vi "PTScanner.set central values.vi"(0 "i ref in":refnum<vi>, 5 "error in(no error)":errorcluster) -> (14 "i ref out":refnum<vi>, 19 "error out":errorcluster)   [LabVIEW 2014, in "PTScanner.lvlib"]
uses:
  PTScanner.lvlib
  CS_Core/CSSystem/CSSystemLib/CSSystemLib.lvlib
  CS_Core/BaseProcess/BaseProcess.lvlib
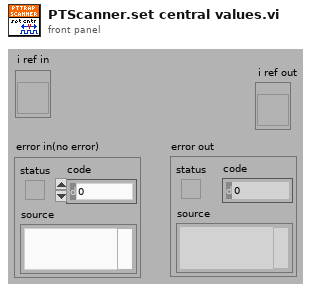
[diagram p1: front panel]
types:
  T1 = typedef "PTScanner.lvlib/PTScanner.i attribute.ctl" = cluster{"Object cmds":T2[], "Steps":cluster{"Finished":bool, "cmd setup":T3[]}[], "curStep":i32, "DIM IDs":cluster{"AllFinished":i32, "Finished":i32, "curStep":i32, "nofSteps":i32, "NomValues":i32[], "1D-Min":i32, "1D-Max":i32, "Dimensions":i32, "MaxDimensions":i32, "ScanedDeviceNames":i32[]}, "All Finished":bool, "DIMs in use":string[], "Running":bool, "Scan Delay":u32, "loop":bool, "Paused":bool, "Formed":bool}
  T2 = typedef "PTScanner.lvlib/PTScanner.obj parameters.ctl" = cluster{"object":string, "DIM address":string, "method":string, "data descriptor":string, "method parameters":cluster{"Name":string, "Descr":string, "Value":string, "Value?":bool}[], "Call Mode":enum16{"Simple DIM", "Synchronous"}, "actValue":dbl, "Centroid":dbl, "Minus Delta":dbl, "Plus Delta":dbl, "increment":dbl, "DIM Status":cluster{"no link":bool, "quality":i32, "Time Stamp":timestamp}, "range":dbl, "DIMChannelIndex":i32}
  T3 = typedef "PTScanner.lvlib/PTScanner.step obj parameters.ctl" = cluster{"obj index":i32, "nomValue":dbl, "fulfilled":bool}
  T4 = cluster{"Name":string, "Descr":string, "Value":string, "Value?":bool}[]
  T5 = typedef "CoreDefs.rawDataType.ctl" = i8[]
  T6 = typedef "CoreDefs.call_type.ctl" = cluster{"Object":string, "Selector":string, "CallType":enum16{"simple", "synchronous", "asynchronous"}, "Async Object":string, "Async Selector":string, "Data Descriptor":T7, "Data":T5, "Error #":i32, "Expire":u32}
  T7 = typedef "BaseProcess.lvlib/BaseProcess.descriptor string definition.ctl" = string
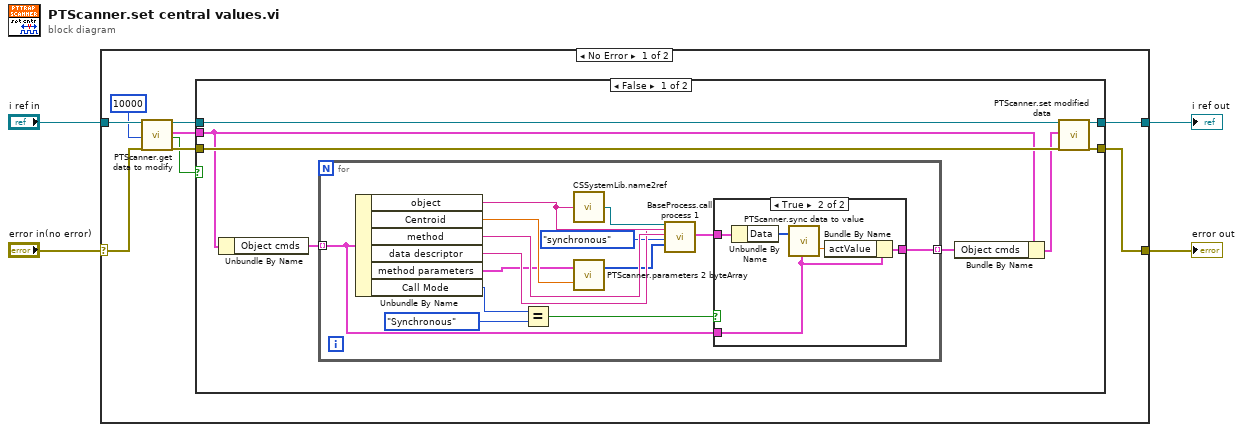
[diagram p0: block diagram]
diagram:
  n1 = case shown="No Error" "error in(no error)" {
    selector: "error in(no error)" -> [w12 w44]
    tunnel: [w8 w44] -> w3
    tunnel: [w9 w45] -> w2
    tunnel: "i ref in" -> [w13 w45]
    frame No Error {
      n2 = call "PTScanner.get data to modify.vi"("i ref in"=w13, "ms timeout (10000)"=10000, "error in (no error)"=w12) -> ("i ref out"=w10:refnum<vi>, "i attribute"=w7:T1, "timed out"=w6:bool, "error out"=w11:errorcluster)  [unwired: 13 in]
      n3 = case shown="False" w6 {
        tunnel: w11 -> [w20 w42]
        tunnel: w10 -> [w19 w43]
        tunnel: [w18 w43] -> w9
        tunnel: [w17 w42] -> w8
        tunnel: w7 -> [w15 _]
        frame False {
          n4 = Unbundle By Name(w15) -> ("Object cmds"=w21:T2[])
          n5 = for {
            tunnel: w21 -> [w22] mode=indexing
            tunnel: [w23] -> w16 mode=indexing
            n6 = Unbundle By Name(w22) -> ("object"=w34:string, "Centroid"=w30:dbl, "method"=w33:string, "data descriptor"=w32:string, "method parameters"=w27:T4, "Call Mode"=w26:enum16{"Simple DIM", "Synchronous"})
            n7 = Equal?(x=w26, y=enum16{"Simple DIM", "Synchronous"}."Synchronous" ("Call Mode")) -> (x = y?=w24:bool)
            n8 = call "CSSystemLib.name2ref.vi"("name"=w34) -> ("obj refnum"=w35:refnum<vi>)
            n9 = call "PTScanner.parameters 2 byteArray.vi"("Parameters"=w27, "nomValue"=w30) -> ("byteArray out"=w29:T5)  [unwired: 17 in]
            n10 = call "BaseProcess.call process 1.vi"("i ref in"=w35, "Object"=w34, "Selector"=w33, "CallType"=enum16{"simple", "synchronous", "asynchronous"}."synchronous", "Data"=w29, "Data Descriptor"=w32) -> ("call cluster out"=w28:T6)  [unwired: 11 in, 2 out]
            n11 = case shown="True" w24 {
              tunnel: w28 -> [_ w41]
              tunnel: [w36 w38] -> w23
              tunnel: w22 -> [w36 w37]
              frame False {
              }
              frame True {
                n12 = Unbundle By Name(w41) -> ("Data"=w40:T5)
                n13 = call "PTScanner.sync data to value.vi"("byteArray"=w40, "obj params"=w37) -> ("actValue"=w39:dbl)  [unwired: 16 in, 1 out]
                n14 = Bundle By Name(cluster=w37, "actValue"=w39) -> (w38:T2)
              }
            }
          }
          n15 = Bundle By Name(cluster=w15, "Object cmds"=w16) -> (w14:T1)
          n16 = call "PTScanner.set modified data.vi"("i ref in"=w19, "CLASS.i attribute"=w14, "error in (no error)"=w20) -> ("i ref out"=w18:refnum<vi>, "error out"=w17:errorcluster)  [unwired: 15 in]
        }
        frame True {
        }
      }
    }
    frame Error {
    }
  }
  "error out" <- w3
  "i ref out" <- w2
